vi "Gradient BG Color.vi"(7 "Number of Rows":i32, 8 "错误输入":errorcluster, 9 "Second BG Color":u32(colorbox), 10 "First BG Color":u32(colorbox), 11 "Listbox Ref":refnum<vi>) -> (0 "错误输出":errorcluster, 3 "Dup Listbox Ref":refnum<vi>)   [LabVIEW 2012, in "Listbox Tool.lvlib"]
uses:
  Listbox Tool.lvlib
  Property/Set and Get Active Row BG Color.vi
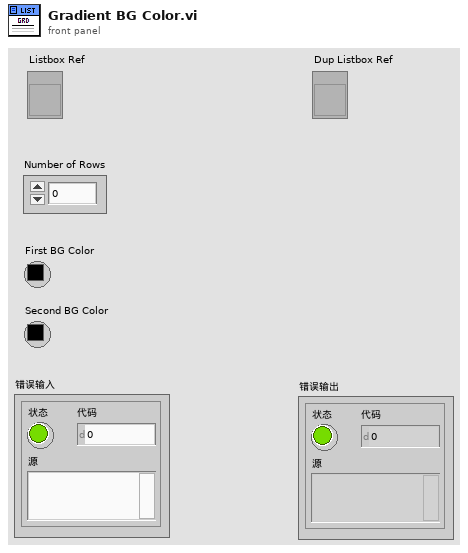
[diagram p1: front panel]
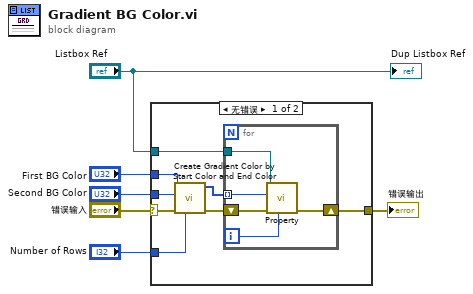
[diagram p0: block diagram]
diagram:
  n1 = case shown="无错误" "错误输入" {
    selector: "错误输入" -> [w11 w20]
    tunnel: [w8 w20] -> w5
    tunnel: "Number of Rows" -> [w12 _]
    tunnel: "First BG Color" -> [w14 _]
    tunnel: "Second BG Color" -> [w13 _]
    tunnel: "Listbox Ref" -> [w7 _]
    frame No Error {
      n2 = call "Create Gradient Color by Start Color and End Color.vi"("错误输入"=w11, "Length"=w12, "End"=w13, "Start"=w14) -> ("错误输出"=w9:errorcluster, "ColorArray"=w10:u32[])  [unwired: 6 in]
      n3 = for {
        tunnel: w10 -> [w15] mode=indexing
        shift-right: [w18] -> w8
        shift-left: w9 -> [w19]
        tunnel: w7 -> [w17]
        i -> [w16]
        n4 = call-poly "Property.vi"("Active Row"=w16, "错误输入"=w19, "CellBG In"=w15, "Listbox Ref"=w17) -> ("错误输出"=w18:errorcluster)  [unwired: 5 in, 2 out]
      }
    }
    frame Error {
    }
  }
  "错误输出" <- w5
  "Dup Listbox Ref" <- "Listbox Ref"
